vi "PROJECT _DETECCION_COLORES_ESP_CAM.vi"() -> ()   [LabVIEW 2021]
uses:
  <vilib>/vision/NI_Vision_Development_Module.lvlib
panel:
  in  "AZUL":i32
  in  "ROJO":i32
  out "AntiRebote":bool
  out "PULSO CONTENDOR LLENO":bool
  out "Counter Red-Elements":dbl
  out "Azul Claro":bool
  out "ROJO":bool
  out "Color Spectrum":dbl[](array[numeric]) format="%.2f"
  in  "Color Sensitivity":u32(ring) items=["Low", "Medium", "High"]
  out "Image":T1(plugin-control)
  in  "stop":bool
  # "ROJO"
  # "AZUL"
  # "DETECCIÓN DE COLOR DESDE ESP32-CAM HACIA LABVIEW\nProf. Dr. David Asiain/ NAOUFAL EL RHAZZALI\nING. MECATRÓNICA/ INSTRUMENTACIÓN AVANZADA"
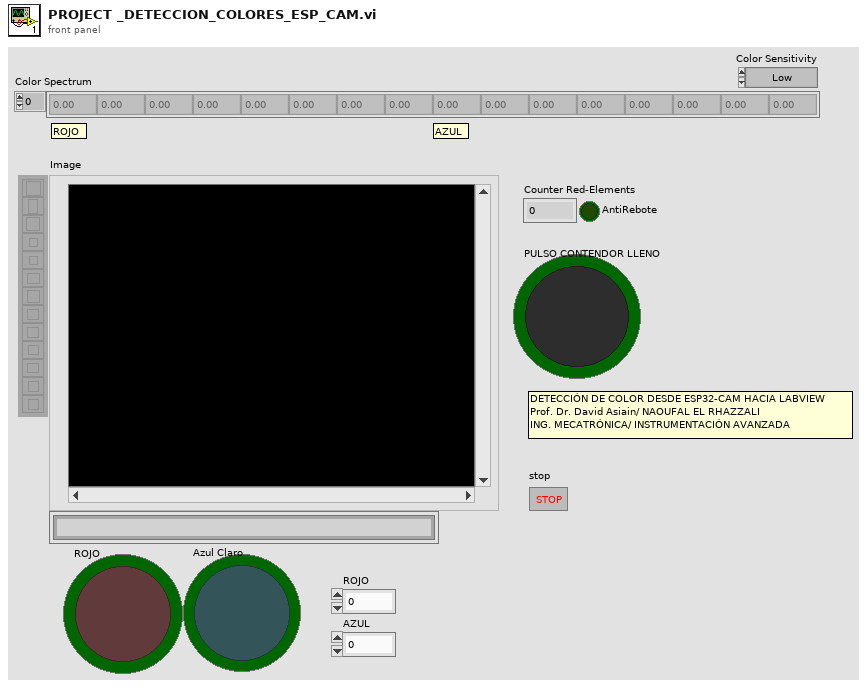
[diagram p1: front panel]
types:
  T1 = typedef "IMAQ Image.ctl" = refnum<image>
  T2 = enum16{"big-endian, network order", "native, host order", "little-endian"}
  T3 = typedef "imagedata.ctl" = cluster{"image type":i32, "image depth":i32, "image":u8[], "mask":u8[], "colors":u32[], "Rectangle":cluster{"left":i16, "top":i16, "right":i16, "bottom":i16}}
  T4 = cluster{"Global Rectangle":i32[], "Contours":cluster{"Contour Type":u32, "ROI Type":u32, "Points":i32[]}[]}
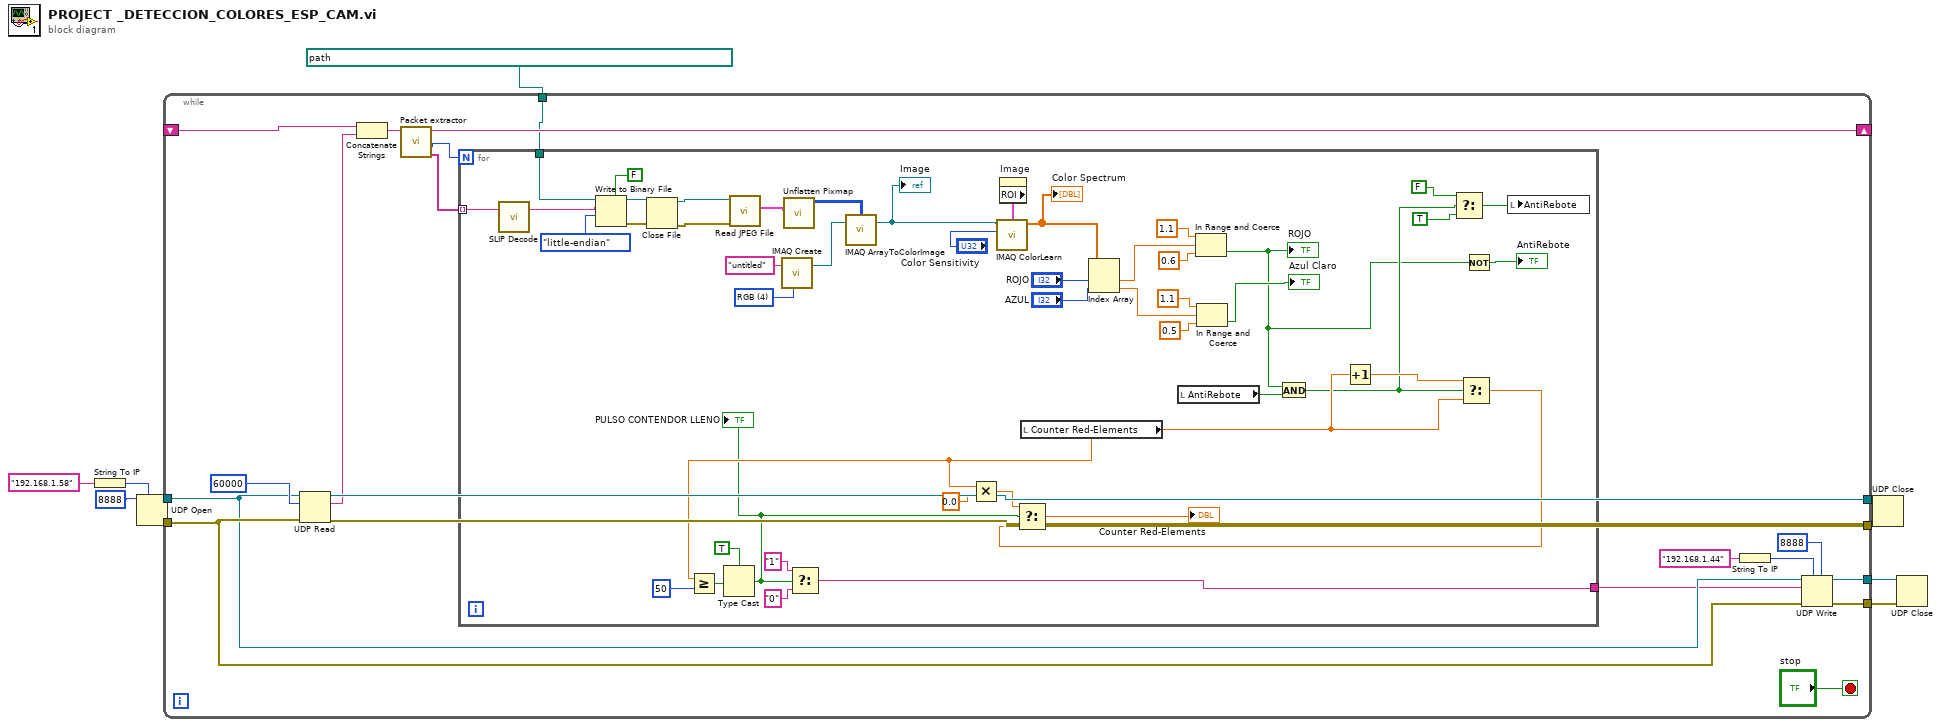
[diagram p0: block diagram]
diagram:
  n1 = String To IP(1:"192.168.1.58" ("name")) -> (0:w5:u32)
  n2 = UDP Open(7:w5, 11:u16 8888 ("port")) -> (port=w10:refnum<k16>, 0:w8:errorcluster)  [unwired: 3 in, 1 out]
  n3 = while {
    tunnel: w10 -> [w19]
    tunnel: [w29] -> w9
    tunnel: w8 -> [w20]
    tunnel: [w28] -> w7
    shift-right: [w26] -> _
    shift-left: _ -> [w25]
    tunnel: [w14] -> w3
    tunnel: path "U:/IngElectrónica/InstrumentacionAvanzadaESP32/LabVIEW/Image/image.jpg" ("file path (use dialog)") -> [w12]
    tunnel: [w11] -> w1
    stop <- "stop" stop-if-true
    n4 = UDP Read(connection ID=w19, max size (548)=60000, 8:w20) -> (data out=w13:string, error out=w28:errorcluster, 3:w29:refnum<k16>)  [unwired: 1 in, 2 out]
    n5 = Concatenate Strings(w25, w13) -> (w22:string)
    n6 = call "Packet extractor.vi"("Buffer in"=w22) -> ("Packets  read"=w23:string[], "N Packetes to read"=w21:i32, "Buffer out"=w26:string)  [unwired: 7 in]
    n7 = for {
      N: w21 -> [_]
      tunnel: w23 -> [w69] mode=indexing
      tunnel: [w48] -> w15
      tunnel: w12 -> [w34]
      w66 = u32 4 items=["8 bits", "16 bits", "Float", "Complex", "RGB", "HSL"] ("Image Type")
      n8 = call "SLIP Decode.vi"("SLIP Input"=w69) -> ("String Output"=w70:string)  [unwired: 1 in, 1 out]
      n9 = Write to Binary File(file (use dialog)=w34, data=w70, 5:FALSE ("prepend array or string size? (T)"), 9:T2."little-endian" ("byte order (0:big-endian, network order)")) -> (refnum out=w74:refnum<file>, error out=w73:errorcluster)  [unwired: 2 in, 1 out]
      n10 = Close File(refnum=w74, error in=w73) -> (path=w75:path, error out=w76:errorcluster)
      n11 = call <vilib>:"Read JPEG File.vi"("error in (no error)"=w76, "path to JPEG file"=w75) -> ("image data"=w33:T3)  [unwired: 7 in, 2 out]
      n12 = call "IMAQ Create"("Image Name"="untitled", "Image Type"=w66) -> ("New Image"=w68:T1)  [unwired: 3 in, 1 out]
      n13 = call <vilib>:"Unflatten Pixmap.vi"("image data"=w33) -> ("24-bit pixmap"=w65:u32[][])  [unwired: 4 in, 6 out]
      n14 = call "IMAQ ArrayToColorImage"("Image Pixels (U32)"=w65, "Image"=w68) -> ("Image Out"=w56:T1)  [unwired: 3 in, 1 out]
      "Image" <- w56
      n15 = property on="Image" class="ImageControl"() -> ("ROI"=w55:T4)  [unwired: 2 in, 2 out]
      n16 = call "IMAQ ColorLearn"("ROI Descriptor"=w55, "Image"=w56, "Color Sensitivity"="Color Sensitivity") -> ("Color Spectrum"=w63:dbl[])  [unwired: 5 in, 1 out]
      "Color Spectrum" <- w63
      n17 = local read "Counter Red-Elements"() -> (w42:dbl)
      n18 = Greater Or Equal?(x=w42, y=50) -> (x >= y?=w53:bool)
      n19 = Type Cast(type=TRUE, x=w53) -> (*(type *) &x=w30:bool)
      "PULSO CONTENDOR LLENO" <- w30
      n20 = Select(t="1", s=w30, f="0") -> (s? t:f=w48:string)
      n21 = Multiply(x=w42, y=0.0) -> (x*y=w47:dbl)
      n22 = Index Array(array=w63, index #1="ROJO", index #2="AZUL") -> (element #1=w62:dbl, element #2=w57:dbl)
      n23 = local read "AntiRebote"() -> (w37:bool)
      n24 = In Range and Coerce(upper limit=1.1, x=w62, lower limit=0.6) -> (In Range?=w31:bool)  [unwired: 1 out]
      "ROJO" <- w31
      n25 = In Range and Coerce(upper limit=1.1, x=w57, lower limit=0.5) -> (In Range?=→"Azul Claro":bool)  [unwired: 1 out]
      n26 = And(x=w31, y=w37) -> (x .and. y?=w32:bool)
      n27 = Increment(x=w42) -> (x+1=w43:dbl)
      n28 = Select(t=FALSE, s=w32, f=TRUE) -> (s? t:f=w39:bool)
      n29 = Select(t=w43, s=w32, f=w42) -> (s? t:f=w45:dbl)
      n30 = Select(t=w47, s=w30, f=w45) -> (s? t:f=→"Counter Red-Elements":dbl)
      n31 = Not(x=w31) -> (.not. x?=→"AntiRebote":bool)
      n32 = local write "AntiRebote"(w39) -> ()
    }
    n33 = String To IP(1:"192.168.1.44" ("name")) -> (0:w18:u32)
    n34 = UDP Write(address=w18, port or service name=u16 8888, connection ID=w19, data in=w15, 8:w20) -> (error out=w14:errorcluster, 3:w11:refnum<k16>)  [unwired: 1 in]
  }
  n35 = UDP Close(connection ID=w9, 8:w7) -> ()  [unwired: 2 out]
  n36 = UDP Close(connection ID=w1, 8:w3) -> ()  [unwired: 2 out]
